vi "base64 decode.vi"(10 "string in (base64-encoded)":string) -> (0 "error out":errorcluster, 2 "string out (decoded)":string)   [LabVIEW 2013]
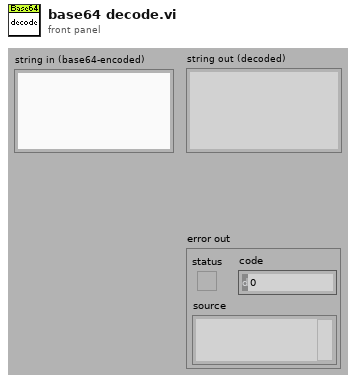
[diagram p1: front panel]
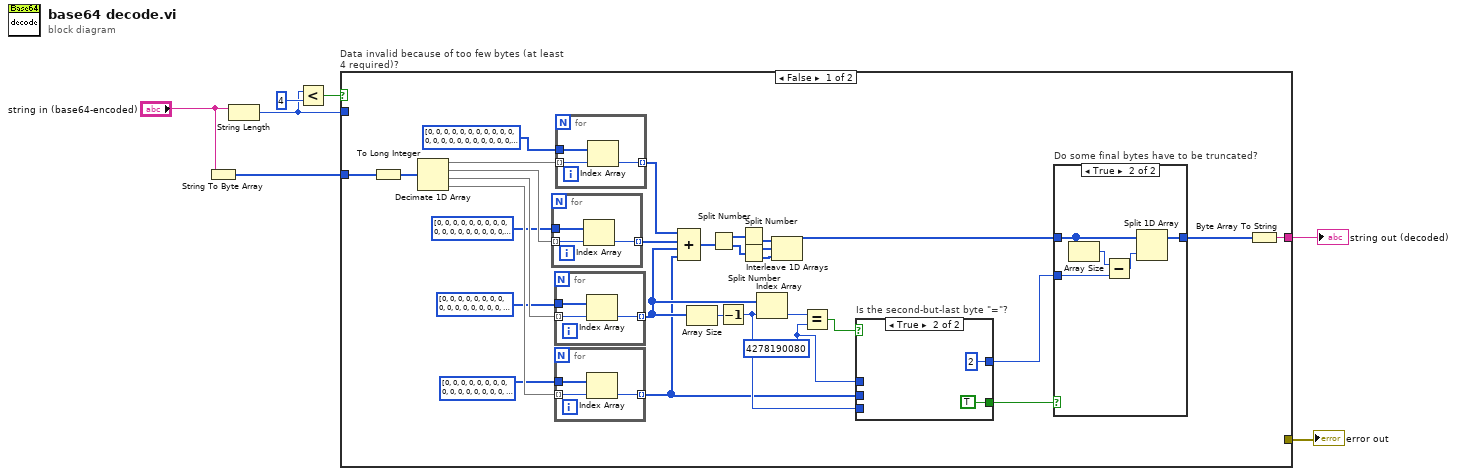
[diagram p0: block diagram]
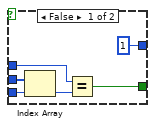
[diagram p3: hidden frame]
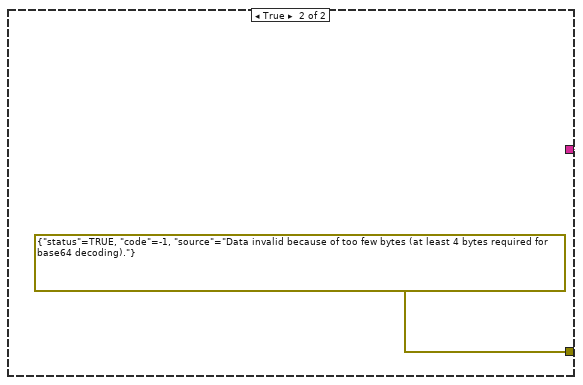
[diagram p4: hidden frame]
diagram:
  n1 = String To Byte Array(string="string in (base64-encoded)") -> (unsigned byte array=w3:u8[])
  n2 = String Length(string="string in (base64-encoded)") -> (length=w1:i32)
  n3 = Less?(x=w1, y=4) -> (x < y?=w2:bool)
  n4 = case "Data invalid because of too few bytes (at least 4 required)?" shown="False" w2 {
    tunnel: w3 -> [w19 _]
    tunnel: [w37 ""] -> w5
    tunnel: w1 -> [_ _]
    tunnel: [_ errorcluster {"status"=TRUE, "code"=-1, "source"="Data invalid because of too few bytes (at least 4 bytes required for base64 decoding)."} ("error IO")] -> w7
    frame False {
      w12 = u32 4278190080 ("y")
      n5 = To Long Integer(number=w19) -> (32bit integer=w36:i32[])
      n6 = Decimate 1D Array(w36) -> (w25:i32[], w35:i32[], w26:i32[], w24:i32[])
      n7 = for {
        tunnel: w35 -> [w59] mode=indexing
        tunnel: u32[] [0, 0, 0, 0, 0, 0, 0, 0, 0, 0, 0, 0, 0, 0, 0, 0, 0, 0, 0, 0, 0, 0, 0, 0, 0, 0, 0, 0, 0, 0, 0, 0, 0, 0, 0, 0, 0, 0, 0, 0, 0, 0, 0, 253952, 0, 0, 0, 258048, 212992, 217088, 221184, 225280, 229376, 233472, 237568, 241664, 245760, 249856, 0, 0, 0, 0, 0, 0, 0, 0, 4096, 8192, 12288, 16384, 20480, 24576, 28672, 32768, 36864, 40960, 45056, 49152, 53248, 57344, 61440, 65536, 69632, 73728, 77824, 81920, 86016, 90112, 94208, 98304, 102400, 0, 0, 0, 0, 0, 0, 106496, 110592, 114688, 118784, 122880, 126976, 131072, 135168, 139264, 143360, 147456, 151552, 155648, 159744, 163840, 167936, 172032, 176128, 180224, 184320, 188416, 192512, 196608, 200704, 204800, 208896, 0, 0, 0, 0, 0, 0, 0, 0, 0, 0, 0, 0, 0, 0, 0, 0, 0, 0, 0, 0, 0, 0, 0, 0, 0, 0, 0, 0, 0, 0, 0, 0, 0, 0, 0, 0, 0, 0, 0, 0, 0, 0, 0, 0, 0, 0, 0, 0, 0, 0, 0, 0, 0, 0, 0, 0, 0, 0, 0, 0, 0, 0, 0, 0, 0, 0, 0, 0, 0, 0, 0, 0, 0, 0, 0, 0, 0, 0, 0, 0, 0, 0, 0, 0, 0, 0, 0, 0, 0, 0, 0, 0, 0, 0, 0, 0, 0, 0, 0, 0, 0, 0, 0, 0, 0, 0, 0, 0, 0, 0, 0, 0, 0, 0, 0, 0, 0, 0, 0, 0, 0, 0, 0, 0, 0, 0, 0, 0, 0, 0, 0, 0, 0] ("array 3") -> [w60]
        tunnel: [w58] -> w33 mode=indexing
        n8 = Index Array(array=w60, index=w59) -> (element=w58:u32)
      }
      n9 = for {
        tunnel: u32[] [0, 0, 0, 0, 0, 0, 0, 0, 0, 0, 0, 0, 0, 0, 0, 0, 0, 0, 0, 0, 0, 0, 0, 0, 0, 0, 0, 0, 0, 0, 0, 0, 0, 0, 0, 0, 0, 0, 0, 0, 0, 0, 0, 3968, 0, 0, 0, 4032, 3328, 3392, 3456, 3520, 3584, 3648, 3712, 3776, 3840, 3904, 0, 0, 0, 4278190080, 0, 0, 0, 0, 64, 128, 192, 256, 320, 384, 448, 512, 576, 640, 704, 768, 832, 896, 960, 1024, 1088, 1152, 1216, 1280, 1344, 1408, 1472, 1536, 1600, 0, 0, 0, 0, 0, 0, 1664, 1728, 1792, 1856, 1920, 1984, 2048, 2112, 2176, 2240, 2304, 2368, 2432, 2496, 2560, 2624, 2688, 2752, 2816, 2880, 2944, 3008, 3072, 3136, 3200, 3264, 0, 0, 0, 0, 0, 0, 0, 0, 0, 0, 0, 0, 0, 0, 0, 0, 0, 0, 0, 0, 0, 0, 0, 0, 0, 0, 0, 0, 0, 0, 0, 0, 0, 0, 0, 0, 0, 0, 0, 0, 0, 0, 0, 0, 0, 0, 0, 0, 0, 0, 0, 0, 0, 0, 0, 0, 0, 0, 0, 0, 0, 0, 0, 0, 0, 0, 0, 0, 0, 0, 0, 0, 0, 0, 0, 0, 0, 0, 0, 0, 0, 0, 0, 0, 0, 0, 0, 0, 0, 0, 0, 0, 0, 0, 0, 0, 0, 0, 0, 0, 0, 0, 0, 0, 0, 0, 0, 0, 0, 0, 0, 0, 0, 0, 0, 0, 0, 0, 0, 0, 0, 0, 0, 0, 0, 0, 0, 0, 0, 0, 0, 0, 0] ("array 2") -> [w57]
        tunnel: [w56] -> w17 mode=indexing
        tunnel: w26 -> [w55] mode=indexing
        n10 = Index Array(array=w57, index=w55) -> (element=w56:u32)
      }
      n11 = for {
        tunnel: u32[] [0, 0, 0, 0, 0, 0, 0, 0, 0, 0, 0, 0, 0, 0, 0, 0, 0, 0, 0, 0, 0, 0, 0, 0, 0, 0, 0, 0, 0, 0, 0, 0, 0, 0, 0, 0, 0, 0, 0, 0, 0, 0, 0, 62, 0, 0, 0, 63, 52, 53, 54, 55, 56, 57, 58, 59, 60, 61, 0, 0, 0, 4278190080, 0, 0, 0, 0, 1, 2, 3, 4, 5, 6, 7, 8, 9, 10, 11, 12, 13, 14, 15, 16, 17, 18, 19, 20, 21, 22, 23, 24, 25, 0, 0, 0, 0, 0, 0, 26, 27, 28, 29, 30, 31, 32, 33, 34, 35, 36, 37, 38, 39, 40, 41, 42, 43, 44, 45, 46, 47, 48, 49, 50, 51, 0, 0, 0, 0, 0, 0, 0, 0, 0, 0, 0, 0, 0, 0, 0, 0, 0, 0, 0, 0, 0, 0, 0, 0, 0, 0, 0, 0, 0, 0, 0, 0, 0, 0, 0, 0, 0, 0, 0, 0, 0, 0, 0, 0, 0, 0, 0, 0, 0, 0, 0, 0, 0, 0, 0, 0, 0, 0, 0, 0, 0, 0, 0, 0, 0, 0, 0, 0, 0, 0, 0, 0, 0, 0, 0, 0, 0, 0, 0, 0, 0, 0, 0, 0, 0, 0, 0, 0, 0, 0, 0, 0, 0, 0, 0, 0, 0, 0, 0, 0, 0, 0, 0, 0, 0, 0, 0, 0, 0, 0, 0, 0, 0, 0, 0, 0, 0, 0, 0, 0, 0, 0, 0, 0, 0, 0, 0, 0, 0, 0, 0, 0, 0] ("Array") -> [w54]
        tunnel: [w53] -> w15 mode=indexing
        tunnel: w24 -> [w52] mode=indexing
        n12 = Index Array(array=w54, index=w52) -> (element=w53:u32)
      }
      n13 = for {
        tunnel: w25 -> [w62] mode=indexing
        tunnel: u32[] [0, 0, 0, 0, 0, 0, 0, 0, 0, 0, 0, 0, 0, 0, 0, 0, 0, 0, 0, 0, 0, 0, 0, 0, 0, 0, 0, 0, 0, 0, 0, 0, 0, 0, 0, 0, 0, 0, 0, 0, 0, 0, 0, 16252928, 0, 0, 0, 16515072, 13631488, 13893632, 14155776, 14417920, 14680064, 14942208, 15204352, 15466496, 15728640, 15990784, 0, 0, 0, 0, 0, 0, 0, 0, 262144, 524288, 786432, 1048576, 1310720, 1572864, 1835008, 2097152, 2359296, 2621440, 2883584, 3145728, 3407872, 3670016, 3932160, 4194304, 4456448, 4718592, 4980736, 5242880, 5505024, 5767168, 6029312, 6291456, 6553600, 0, 0, 0, 0, 0, 0, 6815744, 7077888, 7340032, 7602176, 7864320, 8126464, 8388608, 8650752, 8912896, 9175040, 9437184, 9699328, 9961472, 10223616, 10485760, 10747904, 11010048, 11272192, 11534336, 11796480, 12058624, 12320768, 12582912, 12845056, 13107200, 13369344, 0, 0, 0, 0, 0, 0, 0, 0, 0, 0, 0, 0, 0, 0, 0, 0, 0, 0, 0, 0, 0, 0, 0, 0, 0, 0, 0, 0, 0, 0, 0, 0, 0, 0, 0, 0, 0, 0, 0, 0, 0, 0, 0, 0, 0, 0, 0, 0, 0, 0, 0, 0, 0, 0, 0, 0, 0, 0, 0, 0, 0, 0, 0, 0, 0, 0, 0, 0, 0, 0, 0, 0, 0, 0, 0, 0, 0, 0, 0, 0, 0, 0, 0, 0, 0, 0, 0, 0, 0, 0, 0, 0, 0, 0, 0, 0, 0, 0, 0, 0, 0, 0, 0, 0, 0, 0, 0, 0, 0, 0, 0, 0, 0, 0, 0, 0, 0, 0, 0, 0, 0, 0, 0, 0, 0, 0, 0, 0, 0, 0, 0, 0, 0] ("array 4") -> [w63]
        tunnel: [w61] -> w34 mode=indexing
        n14 = Index Array(array=w63, index=w62) -> (element=w61:u32)
      }
      n15 = Compound Arithmetic op=ADD(w34, w33, w17, w15) -> (w31:u32[])
      n16 = Array Size(array=w17) -> (size(s)=w18:i32)
      n17 = Split Number(x=w31) -> (hi(x)=w32:u16[], lo(x)=w30:u16[])
      n18 = Decrement(x=w18) -> (x-1=w16:i32)
      n19 = Split Number(x=w32) -> (lo(x)=w27:u8[])  [unwired: 1 out]
      n20 = Split Number(x=w30) -> (hi(x)=w28:u8[], lo(x)=w29:u8[])
      n21 = Index Array(array=w17, index=w16) -> (element=w14:u32)
      n22 = Interleave 1D Arrays(w27, w28, w29) -> (w9:u8[])
      n23 = Equal?(x=w14, y=w12) -> (x = y?=w13:bool)
      n24 = case "Is the second-but-last byte \"=\"?" shown="True" w13 {
        tunnel: w16 -> [w49 _]
        tunnel: w15 -> [w48 _]
        tunnel: w12 -> [w46 _]
        tunnel: [w45 TRUE] -> w11
        tunnel: [1 2] -> w10
        frame False {
          n25 = Index Array(array=w48, index=w49) -> (element=w47:u32)
          n26 = Equal?(x=w46, y=w47) -> (x = y?=w45:bool)
        }
        frame True {
        }
      }
      n27 = case "Do some final bytes have to be truncated?" shown="True" w11 {
        tunnel: w10 -> [_ w43]
        tunnel: w9 -> [w38 w39]
        tunnel: [w38 w41] -> w8
        frame False {
        }
        frame True {
          n28 = Array Size(array=w39) -> (size(s)=w40:i32)
          n29 = Subtract(x=w40, y=w43) -> (x-y=w42:i32)
          n30 = Split 1D Array(array=w39, index=w42) -> (first subarray=w41:u8[])  [unwired: 1 out]
        }
      }
      n31 = Byte Array To String(unsigned byte array=w8) -> (string=w37:string)
    }
    frame True {
    }
  }
  "error out" <- w7
  "string out (decoded)" <- w5
